vi "Config Drive Pipeline Command.vi"(8 "Command Info In":T1, 10 "Drive Conditions":cluster{"Field Centric":bool, "Reef Align":bool}) -> (0 "Command Info Out":T1)   [LabVIEW 2023]
uses:
  <vilib>/Rock Robotics/WPI/Framework/Command Status Info.ctl
  <vilib>/Rock Robotics/WPI/Framework/Completion Status.ctl
  <vilib>/Rock Robotics/WPI/Framework/Completion Notifier.ctl
  Framework/Robot Global Data.vi
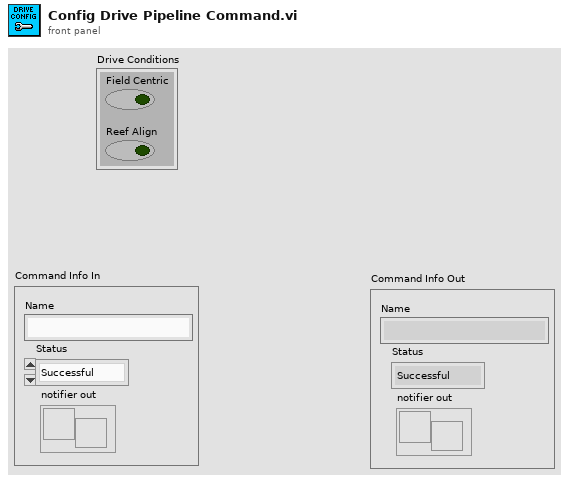
[diagram p1: front panel]
types:
  T1 = typedef "Command Status Info.ctl" = cluster{"Name":string, "Status":T2, "notifier out":T3}
  T2 = typedef "Completion Status.ctl" = enum16{"Successful", "Aborted", "Incomplete"}
  T3 = typedef "Completion Notifier.ctl" = refnum<notifier>
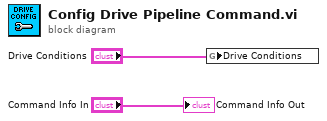
[diagram p0: block diagram]
diagram:
  n1 = global write "Robot Global Data.vi" "Drive Conditions"("Drive Conditions") -> ()
  "Command Info Out" <- "Command Info In"
